vi "Valvulas_On_Off.vi"() -> ()   [LabVIEW 2020]
panel:
  out "Valvulas":T1
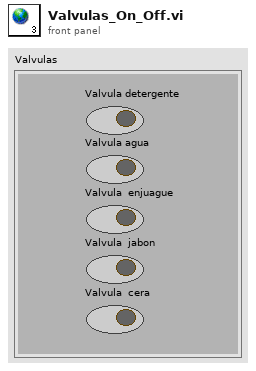
[diagram p1: front panel]
types:
  T1 = cluster{"Valvula detergente":bool, "Valvula agua":bool, "Valvula  enjuague":bool, "Valvula  jabon":bool, "Valvula  cera":bool}
diagram:
